vi "Motor-Setup.vi"(2 "Acc":dbl=1.0, 3 "Velocidade":sgl=0.4, 4 "error":errorcluster, 5 "MG17Motor A":refnum<k7>) -> (0 "error out":errorcluster, 1 "MG17Motor out":refnum<k7>)   [LabVIEW 2014]
doc: "André Romero - 2010\nandretec@ifsc.usp.br\nIFSC - USP"
panel:
  in  "lGearBoxRatio":i32=512
  in  "lStepsPerRev":i32=67
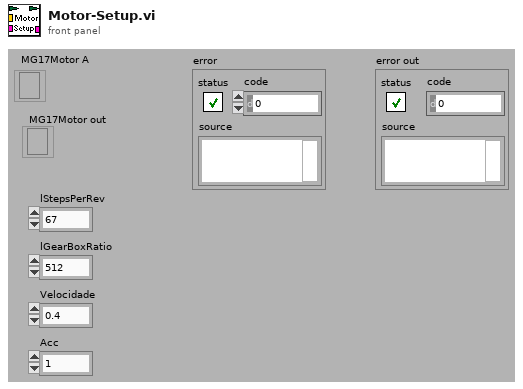
[diagram p1: front panel]
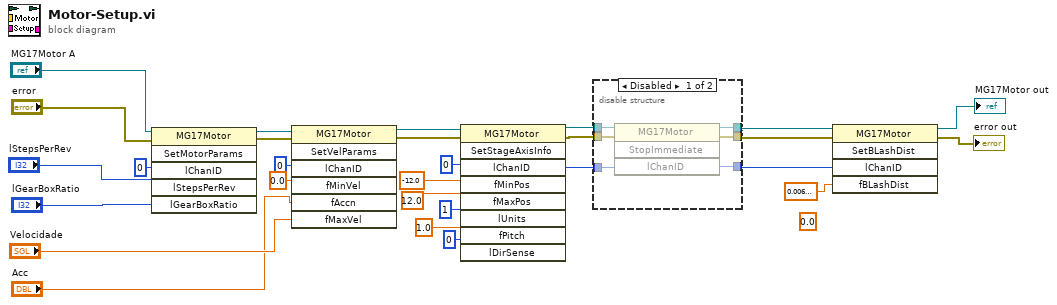
[diagram p0: block diagram]
diagram:
  (unwired) sgl 0.0 ("fBLashDist")
  n1 = invoke class="MG17Motor" method="SetMotorParams"(reference="MG17Motor A", error in="error", "lChanID"=0, "lStepsPerRev"="lStepsPerRev", "lGearBoxRatio"="lGearBoxRatio") -> (reference out=w23:refnum<k7>, error out=w22:errorcluster)  [unwired: 1 in, 4 out]
  n2 = invoke class="MG17Motor" method="SetVelParams"(reference=w23, error in=w22, "lChanID"=0, "fMinVel"=sgl 0.0, "fAccn"="Acc", "fMaxVel"="Velocidade") -> (reference out=w19:refnum<k7>, error out=w18:errorcluster)  [unwired: 1 in, 5 out]
  n3 = invoke class="MG17Motor" method="SetStageAxisInfo"(reference=w19, error in=w18, "lChanID"=0, "fMinPos"=sgl -12.0, "fMaxPos"=sgl 12.0, "lUnits"=1, "fPitch"=sgl 1.0, "lDirSense"=0) -> (reference out=w9:refnum<k7>, error out=w8:errorcluster, "lChanID"=w2:i32)  [unwired: 1 in, 6 out]
  n4 = disable-structure shown="Disabled" {
    disable-tunnel: w9 -> [w34 w37]
    disable-tunnel: w8 -> [w33 w36]
    disable-tunnel: [w32 w37] -> w7
    disable-tunnel: [w31 w36] -> w6
    disable-tunnel: [w30 w35] -> w3
    disable-tunnel: w2 -> [w29 w35]
    frame Disabled {
      n5 = invoke class="MG17Motor" method="StopImmediate"(reference=w34, error in=w33, "lChanID"=w29) -> (reference out=w32:refnum<k7>, error out=w31:errorcluster, "lChanID"=w30:i32)  [unwired: 1 in, 1 out]
    }
    frame Enabled {
    }
  }
  n6 = invoke class="MG17Motor" method="SetBLashDist"(reference=w7, error in=w6, "lChanID"=w3, "fBLashDist"=sgl 0.006) -> (reference out=→"MG17Motor out":refnum<k7>, error out=→"error out":errorcluster)  [unwired: 1 in, 3 out]
